vi "Data_base_server.vi"(0 "Raw Data Pathname":path, 1 "Results File Pathname":path, 3 "Clients time":dbl, 4 "Start time":dbl, 5 "End time":dbl, 6 "Average Meas Time (min)":dbl=100.0 format="%.1f", 7 "Channels from Client":string[][](array[string])=[["Data Base:Measurement:Type", "LDA & Cw"], ["Data Base:Position:No of Inst", "2"], ["Data Base:Position:X1", "-60"], ["Data Base:Position:X2", ""], ["Data Base:Position:Y1", "2"], ["Data Base:Position:Y2", "0.00"], ["Data Base:Position:Z1", "0.00"], ["Data Base:Position:Z2", "2.00"]], 8 "Average Sampling freq":sgl=100.0 format="%.1f", 9 "Rig Name":string) -> (14 "Channel names":string[](array[string])=["Data Base:DB:Filename", "Data Base:Start:Date", "Data Base:Start:Time", "EnFlo Tun:Job: Name", "EnFlo Tun:User: Name", "Data Base:Results:Folder", "Data Base:Results:Filename", "Data Base:Measurement:Type", "Data Base:X Axis:Max", "Data Base:X Axis:Min", "Data Base:Y Axis:Max", "Data Base:Y Axis:Min", "Data Base:Z Axis:Max", "Data Base:Z Axis:Min", "Data Base:No of:Measurements", "Data Base:Av Meas:Frequency (Hz)", "Data Base:Av Meas:Time (min)", "EnFlo Tun:labstrat1:Delta T", "EnFlo Tun:Heater Temp:Average", "EnFlo Tun:Inside:Velocity", "EnFlo Tun:Vorticity: Generators", "EnFlo Tun:Barrier Wall: Height", "EnFlo Tun:Roughness: Height", "EnFlo Tun:Side Wall: Separation", "EnFlo Tun:Obstacle/:Building", "EnFlo Tun:Obstacle: Orientation", "GMU:Source: Type", "GMU:Source: Height", "GMU:Release: Orientation", "GMU:Source:Meas Q", "GMU:Source:Meas Strength", "GMU:Trace: Gas", "GMU:Carrier: Gas", "GMU:Source:Release Temp", "GMU:Suction:Meas Q"], 15 "Channel values":string[](array[string])=["1999:May_1999:G3_3 HD_00006", "13/5/99", "1:55 pm", "National Power", "Paul Hayden", "BMT", "default", "LDA, Cw", "100.00", "-60.00", "2.00", "0.00", "0.00", "0.00", "10", "100.00", "100.00", "1.42", "26.63", "1.54", "\"7 quarter elipticals, 1 metre tall\"", "150mm", "20mm", "No sidewalls installed", "National Power Building", "30 deg", "D=17.5mm", "150 mm", "Vertical", "", "", "Ethane", "48% N2 in He", "", ""], 17 "spreadsheet string":string)   [LabVIEW 2015]
doc: "This is an example of using features of the VI Server as a client. It shows how you might browse from one or more applications that may be exporting data from one or more data stations. \n\nThe example shows how to query a server for its list of exported VIs, how to get references to the VIs, and how call them with the Call By Reference function."
uses:
  ADAM_Global.vi
  Sub VI's/Exp conditions/EnFlo_Tun_Setup_global.vi
  Anemometry/Anemometry Sub Vis/Globals/Constants_global.vi
panel:
  out "Output Array":string[][](array[string])
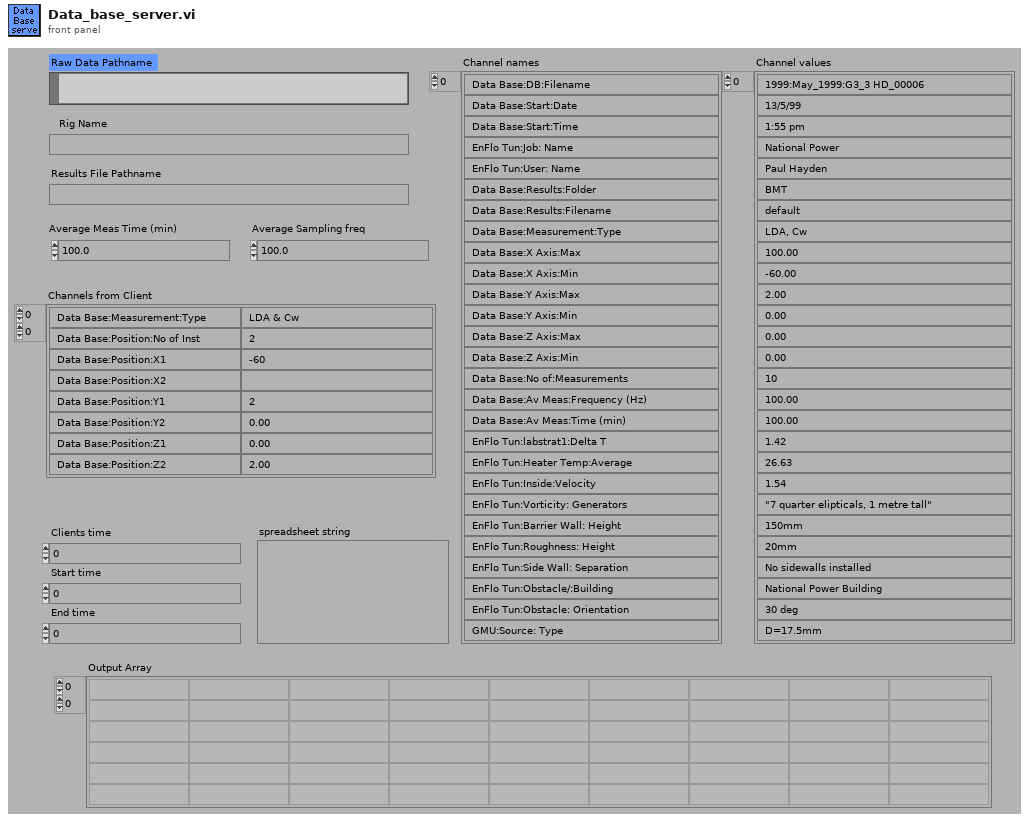
[diagram p1: front panel]
types:
  T1 = cluster{"second":i32, "minute":i32, "hour":i32, "day of month":i32, "month":i32, "year":i32, "day of week":i32, "day of year":i32, "is DST":i32}
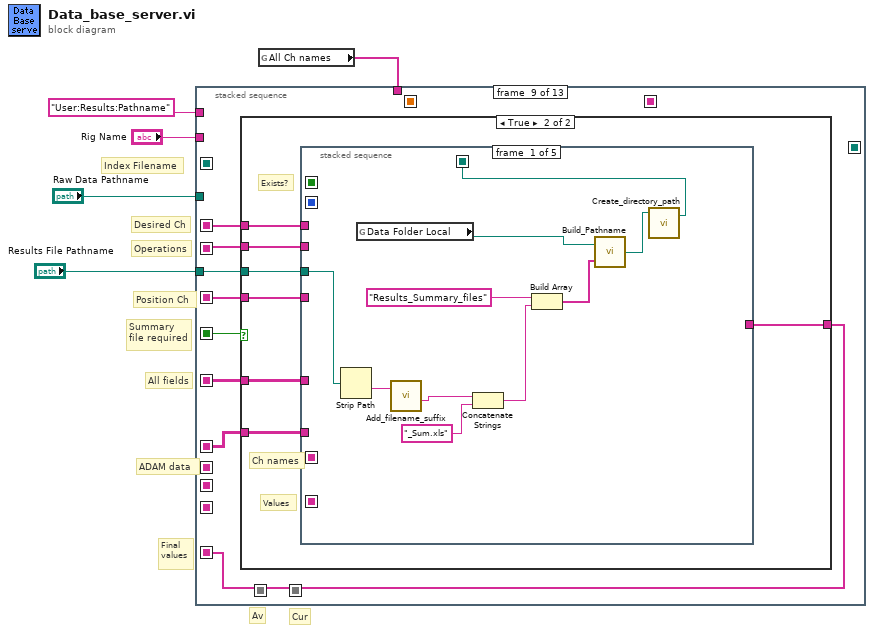
[diagram p0: block diagram]
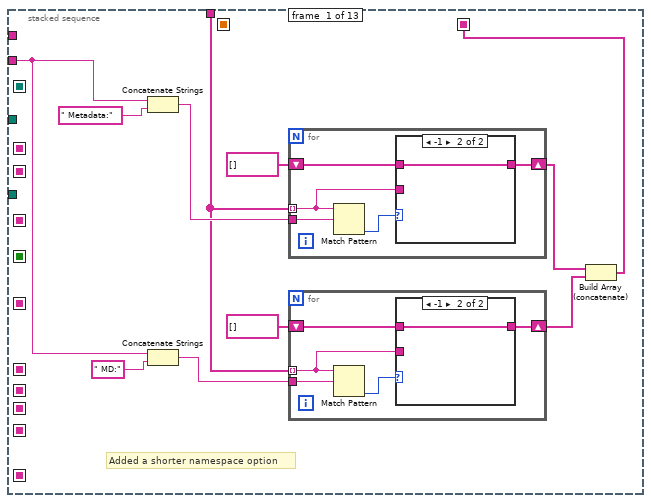
[diagram p2: hidden frame]
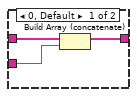
[diagram p3: hidden frame]
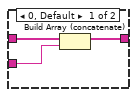
[diagram p4: hidden frame]
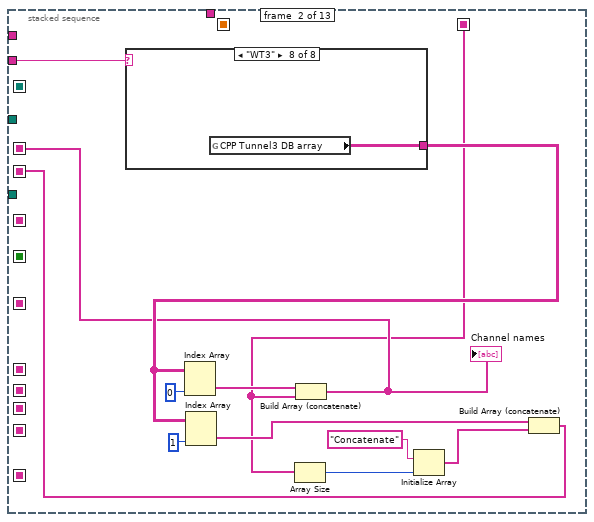
[diagram p5: hidden frame]
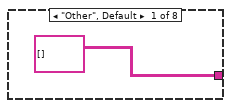
[diagram p6: hidden frame]
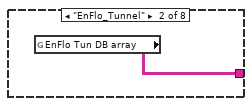
[diagram p7: hidden frame]
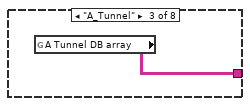
[diagram p8: hidden frame]
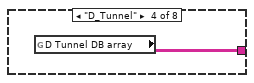
[diagram p9: hidden frame]
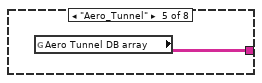
[diagram p10: hidden frame]
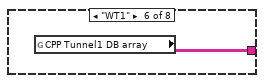
[diagram p11: hidden frame]
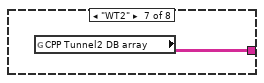
[diagram p12: hidden frame]
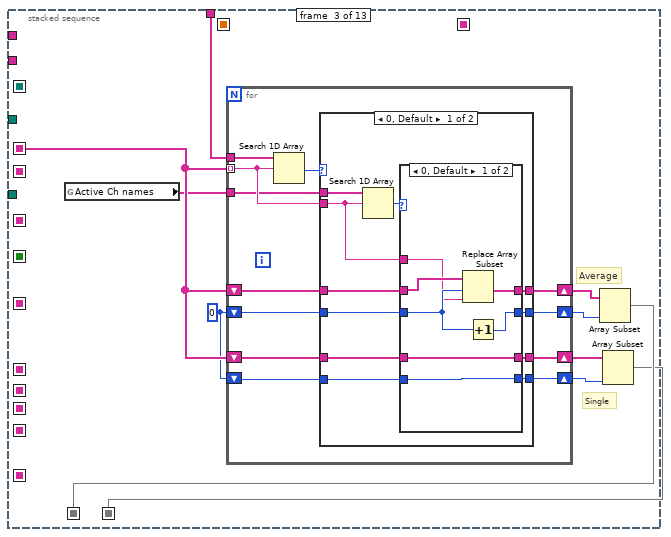
[diagram p13: hidden frame]
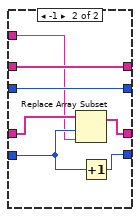
[diagram p14: hidden frame]
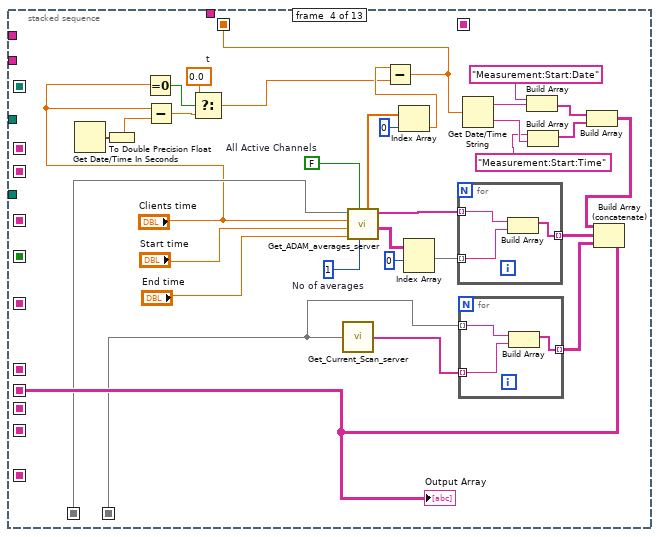
[diagram p16: hidden frame]
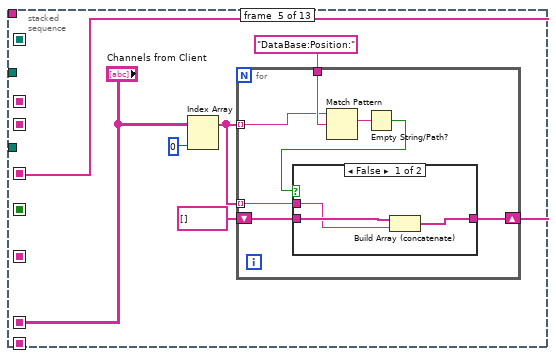
[diagram p17: hidden frame]
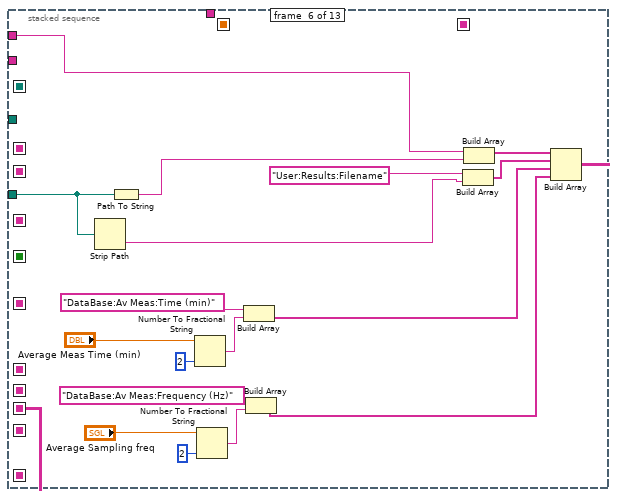
[diagram p19: hidden frame]
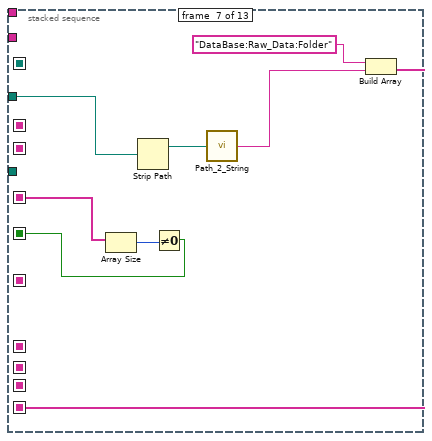
[diagram p20: hidden frame]
diagram:
  # "Cur"
  # "Av"
  # "Index Filename"
  # "Desired Ch"
  # "Operations"
  # "Final\nvalues"
  # "Summary\nfile required"
  # "Position Ch"
  # "All fields"
  # "ADAM data"
  n1 = global read "ADAM_Global.vi" "All Ch names"() -> (w3:string[])
  n2 = stacked-sequence {
    seq-local: [_ w41 _ _ _ _ _ _ _ _ _ _ _] -> [_ _ w64 _ _ _ _ _ w197 _ _ w331 w343]
    seq-local: [_ _ _ w126 _ _ _ _ _ _ _ _ _] -> [_ _ _ _ _ _ _ w191 _ _ _ _ _]
    seq-local: [_ _ _ _ _ w178 _ _ _ _ _ _ _] -> [_ _ _ _ _ _ _ w190 _ _ _ _ _]
    seq-local: [_ _ _ _ _ _ _ w187 _ _ _ _ _] -> [_ _ _ _ _ _ _ _ w195 w293 _ _ _]
    seq-local: [_ _ _ _ _ _ w182 _ _ _ _ _ _] -> [_ _ _ _ _ _ _ w189 _ _ _ _ _]
    seq-local: [_ _ _ _ _ _ _ _ w199 _ _ _ _] -> [_ _ _ _ _ _ _ _ _ w300 _ w332 w342]
    seq-local: [_ _ _ _ w145 _ _ _ _ _ _ _ _] -> [_ _ _ _ _ _ w185 _ w196 _ _ _ _]
    seq-local: [_ _ _ _ "Channels from Client" _ _ _ _ _ _ _ _] -> [_ _ _ _ _ _ _ w188 w192 _ _ _ _]
    seq-local: [_ _ _ _ _ _ w183 _ _ _ _ _ _] -> [_ _ _ _ _ _ _ _ w198 _ _ _ _]
    seq-local: [_ w35 _ _ _ _ _ _ _ _ _ _ _] -> [_ _ _ _ _ _ _ _ w194 _ _ _ _]
    seq-local: [_ _ _ w107 _ _ _ _ _ _ _ _ _] -> [_ _ _ _ _ _ _ _ _ _ _ _ _]
    seq-local: [_ _ _ _ _ _ _ _ _ _ w317 _ _] -> [_ _ _ _ _ _ _ _ _ _ _ w329 w335]
    seq-local: [_ _ w57 _ _ _ _ _ _ _ _ _ _] -> [_ _ _ w118 _ _ _ _ _ _ _ _ _]
    seq-local: [_ _ w56 _ _ _ _ _ _ _ _ _ _] -> [_ _ _ w117 _ _ _ _ _ _ _ _ _]
    seq-local: [w6 _ _ _ _ _ _ _ _ _ _ _ _] -> [_ w38 _ _ _ _ _ _ _ _ _ _ _]
    seq-local: [_ _ _ _ _ _ _ _ _ _ w319 _ _] -> [_ _ _ _ _ _ _ _ _ _ _ _ w334]
    tunnel: "User:Results:Pathname" -> [_ _ _ _ _ w166 _ _ _ _ _ w333 _]
    tunnel: "Results File Pathname" -> [_ _ _ _ _ w163 _ _ w193 _ _ _ _]
    tunnel: "Rig Name" -> [w10 w43 _ _ _ _ _ _ _ w286 w326 _ _]
    tunnel: w3 -> [w11 _ w55 _ _ _ _ _ _ _ _ _ _]
    tunnel: "Raw Data Pathname" -> [_ _ _ _ _ _ w181 _ _ _ _ _ _]
    frame #0 {
      # "Added a shorter namespace option"
      n3 = Concatenate Strings(w10, " Metadata:") -> (w15:string)
      n4 = Concatenate Strings(w10, " MD:" ("string")) -> (w12:string)
      n5 = for {
        tunnel: w15 -> [w27]
        shift-right: [w28] -> w7
        shift-left: string[] [] -> [w29]
        tunnel: w11 -> [w26] mode=indexing
        n6 = Match Pattern(string=w26, regular expression=w27) -> (offset past match=w30:i32)  [unwired: 4 out]
        n7 = case shown="-1" w30 {
          tunnel: w29 -> [w33 w34]
          tunnel: [w31 w34] -> w28
          tunnel: w26 -> [w32 _]
          frame 0, Default {
            n8 = Build Array (concatenate)(w33, w32) -> (w31:string[])
          }
          frame -1 {
          }
        }
      }
      n9 = for {
        tunnel: w12 -> [w18]
        shift-right: [w19] -> w8
        shift-left: string[] [] -> [w20]
        tunnel: w11 -> [w17] mode=indexing
        n10 = Match Pattern(string=w17, regular expression=w18) -> (offset past match=w21:i32)  [unwired: 4 out]
        n11 = case shown="-1" w21 {
          tunnel: w20 -> [w24 w25]
          tunnel: [w22 w25] -> w19
          tunnel: w17 -> [w23 _]
          frame 0, Default {
            n12 = Build Array (concatenate)(w24, w23) -> (w22:string[])
          }
          frame -1 {
          }
        }
      }
      n13 = Build Array (concatenate)(w7, w8) -> (w6:string[])
    }
    frame #1 {
      n14 = case shown="\"WT3\"" w43 {
        tunnel: [string[][] [] ("EnFlo Tun DB array") w48 w49 w50 w51 w52 w53 w54] -> w44
        frame "Other", Default {
        }
        frame "EnFlo_Tunnel" {
          n15 = global read "EnFlo_Tun_Setup_global.vi" "EnFlo Tun DB array"() -> (w48:string[][])
        }
        frame "A_Tunnel" {
          n16 = global read "EnFlo_Tun_Setup_global.vi" "A Tunnel DB array"() -> (w49:string[][])
        }
        frame "D_Tunnel" {
          n17 = global read "EnFlo_Tun_Setup_global.vi" "D Tunnel DB array"() -> (w50:string[][])
        }
        frame "Aero_Tunnel" {
          n18 = global read "EnFlo_Tun_Setup_global.vi" "Aero Tunnel DB array"() -> (w51:string[][])
        }
        frame "WT1" {
          n19 = global read "EnFlo_Tun_Setup_global.vi" "CPP Tunnel1 DB array"() -> (w52:string[][])
        }
        frame "WT2" {
          n20 = global read "EnFlo_Tun_Setup_global.vi" "CPP Tunnel2 DB array"() -> (w53:string[][])
        }
        frame "WT3" {
          n21 = global read "EnFlo_Tun_Setup_global.vi" "CPP Tunnel3 DB array"() -> (w54:string[][])
        }
      }
      n22 = Index Array(array=w44, index (col)=0) -> (element=w42:string[])  [unwired: 1 in]
      n23 = Index Array(array=w44, index (col)=1) -> (element=w40:string[])  [unwired: 1 in]
      n24 = Array Size(array=w38) -> (size(s)=w39:i32)
      n25 = Build Array (concatenate)(w42, w38) -> (w41:string[])
      "Channel names" <- w41
      n26 = Initialize Array("Concatenate", w39) -> (w36:string[])
      n27 = Build Array (concatenate)(w40, w36) -> (w35:string[])
    }
    frame #2 {
      w62 = 0
      # "Single"
      # "Average"
      n28 = global read "ADAM_Global.vi" "Active Ch names"() -> (w63:string[])
      n29 = for {
        tunnel: w64 -> [w70] mode=indexing
        tunnel: w55 -> [w76]
        shift-right: [w74] -> w61
        shift-left: w64 -> [w73]
        shift-right: [w72] -> w59
        shift-left: w64 -> [w71]
        tunnel: w63 -> [w69]
        shift-right: [w65] -> w60
        shift-left: w62 -> [w66]
        shift-right: [w67] -> w58
        shift-left: w62 -> [w68]
        n30 = Search 1D Array(1D array=w76, element=w70) -> (index of element=w75:i32)  [unwired: 1 out]
        n31 = case shown="0, Default" w75 {
          tunnel: [w78 w105] -> w74
          tunnel: w73 -> [w79 w105]
          tunnel: [w84 w104] -> w72
          tunnel: w71 -> [w85 w104]
          tunnel: w70 -> [w77 _]
          tunnel: w69 -> [w87 _]
          tunnel: w68 -> [w83 w102]
          tunnel: [w82 w102] -> w67
          tunnel: w66 -> [w81 w103]
          tunnel: [w80 w103] -> w65
          frame 0, Default {
            n32 = Search 1D Array(1D array=w87, element=w77) -> (index of element=w86:i32)  [unwired: 1 out]
            n33 = case shown="0, Default" w86 {
              tunnel: w85 -> [w90 w101]
              tunnel: [w90 w100] -> w84
              tunnel: w83 -> [w89 w99]
              tunnel: [w89 w98] -> w82
              tunnel: w81 -> [w94 w97]
              tunnel: [w91 w97] -> w80
              tunnel: w79 -> [w93 w96]
              tunnel: [w92 w96] -> w78
              tunnel: w77 -> [w88 w95]
              frame 0, Default {
                n34 = Replace Array Subset(array=w93, new element=w88, index=w94) -> (w92:string[])
                n35 = Increment(x=w94) -> (x+1=w91:i32)
              }
              frame -1 {
                n36 = Replace Array Subset(array=w101, new element=w95, index=w99) -> (w100:string[])
                n37 = Increment(x=w99) -> (x+1=w98:i32)
              }
            }
          }
          frame -1 {
          }
        }
      }
      n38 = Array Subset(array=w61, length=w60) -> (w57:string[])  [unwired: 1 in]
      n39 = Array Subset(array=w59, length=w58) -> (w56:string[])  [unwired: 1 in]
    }
    frame #3 {
      w111 = 0.0  # t
      w119 = FALSE  # All Active Channels
      w137 = 1  # No of averages
      n40 = Get Date/Time In Seconds() -> (seconds since 1Jan1904=w106:timestamp)
      n41 = To Double Precision Float(number=w106) -> (double precision float=w114:dbl)
      n42 = Equal To 0?(x="Clients time") -> (x = 0?=w112:bool)
      n43 = Subtract(x="Clients time", y=w114) -> (x-y=w113:dbl)
      n44 = Select(t=w111, s=w112, f=w113) -> (s? t:f=w108:dbl)
      n45 = call "Get_Current_Scan_server.vi"("Desired Channels"=w117) -> ("String values"=w116:string[])  [unwired: 2 out]
      n46 = call "Get_ADAM_averages_server.vi"("No of averages"=w137, "All Active Channels"=w119, "End time"="End time", "Start time"="Start time", "Clients time"="Clients time", "ADAM Ch Names"=w118) -> ("Values"=w122:string[][], "Titles"=w125:string[], "Times"=w135:dbl[])  [unwired: 2 out]
      n47 = Index Array(array=w135, index=0) -> (element=w109:dbl)
      n48 = Subtract(x=w109, y=w108) -> (x-y=w107:dbl)
      n49 = Index Array(array=w122, index (row)=0) -> (element=w124:string[])  [unwired: 1 in]
      n50 = for {
        tunnel: w125 -> [w143] mode=indexing
        tunnel: w124 -> [w142] mode=indexing
        tunnel: [w141] -> w127 mode=indexing
        n51 = Build Array(w143, w142) -> (w141:string[])
      }
      n52 = for {
        tunnel: w116 -> [w140] mode=indexing
        tunnel: [w139] -> w115 mode=indexing
        tunnel: w117 -> [w138] mode=indexing
        n53 = Build Array(w138, w140) -> (w139:string[])
      }
      n54 = Get Date/Time String(seconds (now)=w107) -> (date string=w133:string, time string=w132:string)  [unwired: 2 out]
      n55 = Build Array("Measurement:Start:Date", w133) -> (w130:string[])
      n56 = Build Array("Measurement:Start:Time", w132) -> (w129:string[])
      n57 = Build Array(w130, w129) -> (w128:string[][])
      n58 = Build Array (concatenate)(w128, w127, w115) -> (w126:string[][])
      "Output Array" <- w126
    }
    frame #4 {
      n59 = Index Array(array="Channels from Client", index (col)=0) -> (element=w147:string[])  [unwired: 1 in]
      n60 = for {
        tunnel: "DataBase:Position:" ("String to match") -> [w156]
        tunnel: w147 -> [w155] mode=indexing
        shift-right: [w150] -> w145
        shift-left: string[] [] -> [w151]
        tunnel: w147 -> [w152] mode=indexing
        n61 = Match Pattern(string=w155, regular expression=w156) -> (match substring=w154:string)  [unwired: 4 out]
        n62 = Empty String/Path?(string/path=w154) -> (empty?=w153:bool)
        n63 = case shown="False" w153 {
          tunnel: w152 -> [w157 _]
          tunnel: w151 -> [w159 w160]
          tunnel: [w158 w160] -> w150
          frame False {
            n64 = Build Array (concatenate)(w159, w157) -> (w158:string[])
          }
          frame True {
          }
        }
      }
    }
    frame #5 {
      n65 = Strip Path(path=w163) -> (name=w162:string)  [unwired: 1 out]
      n66 = Path To String(path=w163) -> (string=w165:string)
      n67 = Number To Fractional String(number="Average Meas Time (min)", precision (6)=i16 2) -> (F-format string=w175:string)  [unwired: 2 out]
      n68 = Number To Fractional String(number="Average Sampling freq", precision (6)=i16 2) -> (F-format string=w173:string)  [unwired: 2 out]
      n69 = Build Array("DataBase:Av Meas:Time (min)", w175) -> (w169:string[])
      n70 = Build Array("DataBase:Av Meas:Frequency (Hz)", w173) -> (w168:string[])
      n71 = Build Array("User:Results:Filename", w162) -> (w161:string[])
      n72 = Build Array(w166, w165) -> (w167:string[])
      n73 = Build Array(w167, w161, w169, w168) -> (w178:string[][])
    }
    frame #6 {
      n74 = Array Size(array=w185) -> (size(s)=w184:i32)
      n75 = Strip Path(path=w181) -> (stripped path=w180:path)  [unwired: 1 out]
      n76 = Not Equal To 0?(x=w184) -> (x != 0?=w183:bool)
      n77 = call "Path_2_String.vi"("Real Path"=w180) -> ("Path String"=w179:string)
      n78 = Build Array("DataBase:Raw_Data:Folder", w179) -> (w182:string[])
    }
    frame #7 {
      n79 = Build Array (concatenate)(w188, w191, w190, w189) -> (w187:string[][])
    }
    frame #8 {
      n80 = case shown="True" w198 {
        tunnel: [w201 w213] -> w199
        tunnel: w197 -> [w202 w212]
        tunnel: w196 -> [_ w211]
        tunnel: w195 -> [w203 w210]
        tunnel: w194 -> [_ w209]
        tunnel: w193 -> [_ w208]
        tunnel: w192 -> [_ w207]
        frame False {
          n81 = Index Array(array=w203, index (col)=1) -> (element=w204:string[])  [unwired: 1 in]
          n82 = Index Array(array=w203, index (col)=0) -> (element=w200:string[])  [unwired: 1 in]
          n83 = call "Merge_row_values.vi"("Present Row values"=w204, "Present Channels"=w200, "Desired Channels"=w202) -> ("Desired Row values"=w201:string[])  [unwired: 1 out]
        }
        frame True {
          # "Exists?"
          # "Ch names"
          # "Values"
          n84 = stacked-sequence {
            seq-local: [_ _ w244 _ _] -> [_ _ _ w260 w282]
            seq-local: [_ _ w240 _ _] -> [_ _ _ w264 w284]
            seq-local: [w221 _ _ _ _] -> [_ w227 w242 _ w285]
            seq-local: [_ w224 _ _ _] -> [_ _ w236 _ w283]
            seq-local: [_ _ w237 _ _] -> [_ _ _ _ w281]
            tunnel: [_ _ _ w265 _] -> w213
            tunnel: w212 -> [_ _ w243 w262 _]
            tunnel: w211 -> [_ _ w250 _ _]
            tunnel: w210 -> [_ _ w246 _ _]
            tunnel: w209 -> [_ _ _ w263 _]
            tunnel: w208 -> [w222 _ _ _ _]
            tunnel: w207 -> [_ w230 _ _ _]
            frame #0 {
              n85 = Strip Path(path=w222) -> (name=w215:string)  [unwired: 1 out]
              n86 = global read "Constants_global.vi" "Data Folder Local"() -> (w220:path)
              n87 = call "Add_filename_suffix.vi"("Filename"=w215) -> ("Base name"=w214:string)  [unwired: 1 in, 3 out]
              n88 = Concatenate Strings(w214, "_Sum.xls" ("Substring")) -> (w216:string)
              n89 = Build Array("Results_Summary_files", w216) -> (w219:string[])
              n90 = call "Build_Pathname.vi"("PathElements"=w219, "PathnameIn"=w220) -> ("AppendedPath"=w217:path)
              n91 = call "Create_directory_path.vi"("Path name"=w217) -> ("Path name Out"=w221:path)  [unwired: 2 in, 1 out]
            }
            frame #1 {
              n92 = Index Array(array=w230, index (col)=0) -> (element=w234:string[])  [unwired: 1 in]
              n93 = Search 1D Array(1D array=w234, element="Does the results file already exist?") -> (index of element=w231:i32)  [unwired: 1 out]
              n94 = Index Array(array=w230, index (row)=w231, index (col)=1 ("Index")) -> (element=w229:string)
              n95 = call "Does_file_exist_(simple).vi"("Pathname"=w227) -> ("exists?"=w225:bool)
              n96 = Not Equal?(x="FALSE", y=w229) -> (x != y?=w226:bool)
              n97 = And(x=w225, y=w226) -> (x .and. y?=w224:bool)
            }
            frame #2 {
              n98 = Build Array (concatenate)(w243, w250) -> (w249:string[])
              n99 = case shown="True" w236 {
                tunnel: w249 -> [w253 w259]
                tunnel: w242 -> [_ w258]
                tunnel: [w253 w257] -> w240
                tunnel: [string[][] [] ("Channel Values") w256] -> w238
                tunnel: [0 ("Offset from File End") w255] -> w237
                frame False {
                }
                frame True {
                  n100 = call "Read_Ch_data_file.vi"("Present Channels"=w259, "Output"=enum16{"All Ch data", "The last few rows"}."All Ch data", "Filename"=w258) -> ("Channel Values"=w256:string[][], "Merged Channels"=w257:string[], "Offset from File End"=w255:i32)  [unwired: 2 in, 2 out]
                }
              }
              n101 = Index Array(array=w246, index (col)=1) -> (element=w245:string[])  [unwired: 1 in]
              n102 = Index Array(array=w246, index (col)=0) -> (element=w241:string[])  [unwired: 1 in]
              n103 = call "Merge_row_values.vi"("Present Row values"=w245, "Present Channels"=w241, "Desired Channels"=w240) -> ("Desired Row values"=w239:string[])  [unwired: 1 out]
              n104 = Build Array (concatenate)(w238, w239) -> (w244:string[][])
            }
            frame #3 {
              n105 = call "Average_Column_Values.vi"("Present Values"=w260, "Present Channels"=w264, "Channel operations"=w263, "Channel names for operations"=w262) -> ("Desired Row values"=w261:string[])
              n106 = call "String_to_Pos_array.vi"("Channel values"=w260, "Channel names"=w264) -> ("Positions"=w268:dbl[][], "No of Inst"=w267:i32)
              n107 = while {
                tunnel: [w274] -> w266
                tunnel: w267 -> [w278]
                tunnel: w268 -> [w273]
                i -> [w271]
                stop <- w275 continue-if-true
                w269 = 3 ("x")
                n108 = Increment(x=w271) -> (x+1=w279:i32)
                n109 = Multiply(x=w269, y=w271) -> (x*y=w270:i32)
                n110 = Array Subset(array=w273, index (col)=w270, length (col)=w269) -> (w272:dbl[][])  [unwired: 2 in]
                n111 = call "Cal_Pos_Max_Min.vi"("Positions"=w272) -> ("Position Info"=w274:string[][], "Instrument moved?"=w276:bool)
                n112 = Less?(x=w279, y=w278) -> (x < y?=w277:bool)
                n113 = Compound Arithmetic op=AND(invert w276, w277) -> (w275:bool)
              }
              n114 = call "Replace_Channel_Values.vi"("Channels to replace"=w266, "Present Values"=w261, "Present Channels"=w262) -> ("Merged Row values"=w265:string[])  [unwired: 1 out]
            }
            frame #4 {
              w280 = TRUE  # Append last row only
              n115 = call "Write_Ch_data_file.vi"("Append last row only"=w280, "exists?"=w283, "Write offset fr file end"=w281, "Channel Values"=w282, "Channel names"=w284, "Filename"=w285) -> ()  [unwired: 2 in, 4 out]
            }
          }
        }
      }
    }
    frame #9 {
      n116 = Index Array(array=w293, index (col)=0) -> (element=w297:string[])  [unwired: 1 in]
      n117 = Concatenate Strings(w286, ":Pitot:Velocity" ("Substring")) -> (w299:string)
      n118 = Concatenate Strings(w286, ":Speed:Dem Velocity" ("Substring")) -> (w288:string)
      n119 = Concatenate Strings(w286, ":Speed:Calib Tweak" ("Substring")) -> (w287:string)
      n120 = Build Array(w288, w287, w299) -> (w296:string[])
      n121 = for {
        tunnel: w297 -> [w315]
        tunnel: w296 -> [w314] mode=indexing
        tunnel: [w313] -> w295 mode=indexing
        tunnel: [w312] -> w292 mode=indexing
        n122 = Search 1D Array(1D array=w315, element=w314) -> (index of element=w312:i32)  [unwired: 1 out]
        n123 = Greater Or Equal To 0?(x=w312) -> (x >= 0?=w313:bool)
      }
      n124 = And Array Elements(Boolean array=w295) -> (logical AND=w294:bool)
      n125 = case shown="True" w294 {
        tunnel: w293 -> [_ w306]
        tunnel: w292 -> [_ w304]
        tunnel: w286 -> [_ w302]
        frame False {
        }
        frame True {
          n126 = Index Array(array=w306, index (col)=1) -> (element=w305:string[])  [unwired: 1 in]
          n127 = for {
            tunnel: w305 -> [w311]
            tunnel: w304 -> [w310] mode=indexing
            tunnel: [w308] -> w303 mode=indexing
            n128 = Index Array(array=w311, index=w310) -> (element=w309:string)
            n129 = Fract/Exp String To Number(string=w309) -> (number=w308:dbl)  [unwired: 4 out]
          }
          n130 = call "Add_to_speed_calib_file.vi"("New Row"=w303, "Rig Name"=w302, "Mode"=enum16{"Add Row", "Get Error Value"}."Add Row") -> ()  [unwired: 3 in, 2 out]
        }
      }
      "Channel values" <- w300
    }
    frame #10 {
      n131 = Get Date/Time In Seconds() -> (seconds since 1Jan1904=w316:timestamp)
      n132 = global read "Constants_global.vi" "Data Folder Local"() -> (w321:path)
      n133 = call <vilib>:"LV70TimeStampToDateRec.vi"("time stamp"=w316) -> ("date time rec"=w328:T1)
      n134 = global read "Constants_global.vi" "Data Folder"() -> (w320:path)
      n135 = Unbundle By Name(w328) -> ("year"=w327:i32)
      n136 = Number To Decimal String(number=w327) -> (decimal integer string=w323:string)  [unwired: 1 out]
      n137 = Format Into String(format string="-%s.xls", initial string=w326, w323) -> (resulting string=w325:string)  [unwired: 1 in, 1 out]
      n138 = Build Array(w323, w326, w325) -> (w322:string[])
      n139 = call "Build_Pathname.vi"("PathElements"=w322, "PathnameIn"=w320) -> ("AppendedPath"=w319:path)
      n140 = call "Build_Pathname.vi"("PathElements"=w322, "PathnameIn"=w321) -> ("AppendedPath"=w318:path)
      n141 = call "Create_directory_path.vi"("Path name"=w318) -> ("Path name Out"=w317:path)  [unwired: 2 in, 1 out]
    }
    frame #11 {
      n142 = call "Update_Ch_data_file.vi"("Range"=enum16{"All Ch data", "The last few rows"}."The last few rows", "Channel to search on"=w333, "New Row values"=w332, "Present Channels"=w331, "Filename"=w329) -> ()  [unwired: 2 in, 5 out]
    }
    frame #12 {
      w344 = string[] []
      n143 = for {
        shift-right: [w353] -> w337
        shift-left: w344 -> [w354]
        shift-right: [w355] -> w341
        shift-left: w344 -> [w356]
        tunnel: w342 -> [w352] mode=indexing
        tunnel: w343 -> [w351] mode=indexing
        n144 = Empty String/Path?(string/path=w352) -> (empty?=w357:bool)
        n145 = case shown="True" w357 {
          tunnel: w356 -> [w363 w365]
          tunnel: [w362 w365] -> w355
          tunnel: w354 -> [w361 w364]
          tunnel: [w360 w364] -> w353
          tunnel: w352 -> [w359 _]
          tunnel: w351 -> [w358 _]
          frame False {
            n146 = Build Array (concatenate)(w363, w358) -> (w362:string[])
            n147 = Build Array (concatenate)(w361, w359) -> (w360:string[])
          }
          frame True {
          }
        }
      }
      n148 = for {
        tunnel: w341 -> [w350] mode=indexing
        tunnel: [w349] -> w340 mode=indexing
        tunnel: [w348] -> w339 mode=indexing
        tunnel: [w347] -> w338 mode=indexing
        n149 = call "Split_Ch_name.vi"("Ch name"=w350) -> ("Top level"=w349:string, "Middle"=w348:string, "Low level"=w347:string)
      }
      n150 = call "Updated_File_Copy.vi"("Target Path"=w334, "Source Path"=w335) -> ()  [unwired: 2 out]
      n151 = Build Array(w340, w339, w338, w337) -> (w336:string[][])
      n152 = Array To Spreadsheet String(array=w336, 3:"%s" ("format string")) -> (spreadsheet string=→"spreadsheet string":string)  [unwired: 1 out]
    }
  }
